vi "2 Simple Time.vi"(11 "Timestamp":string) -> (1 "Error?":bool, 3 "Simple Time":i64)   [LabVIEW 2013]
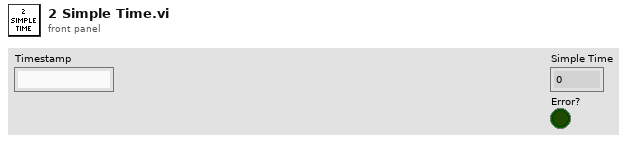
[diagram p1: front panel]
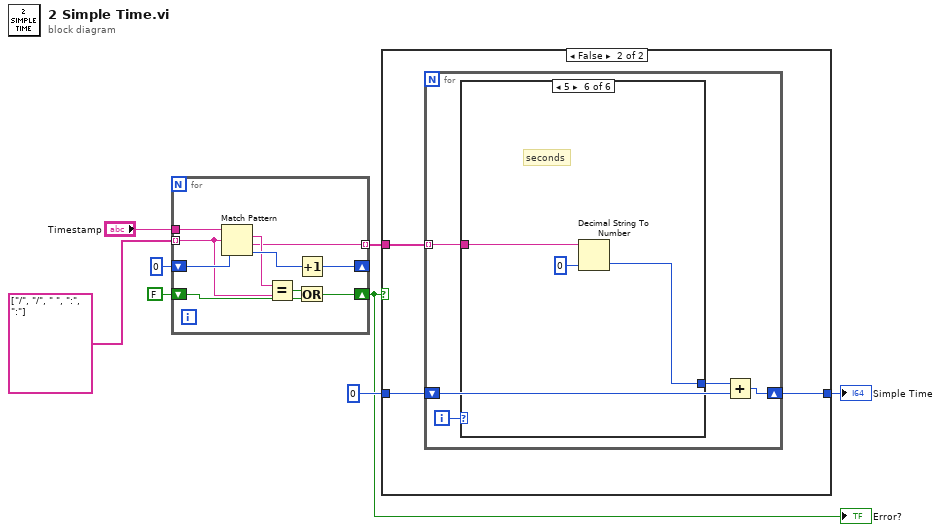
[diagram p0: block diagram]
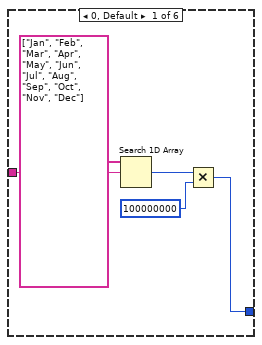
[diagram p3: hidden frame]
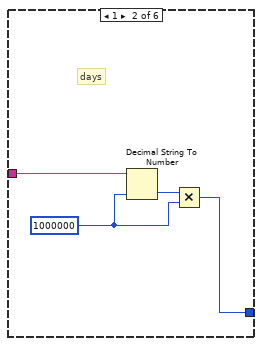
[diagram p4: hidden frame]
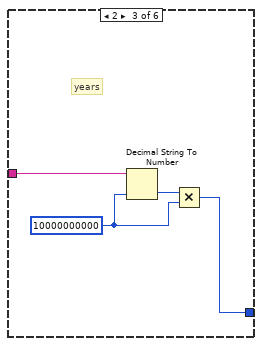
[diagram p5: hidden frame]
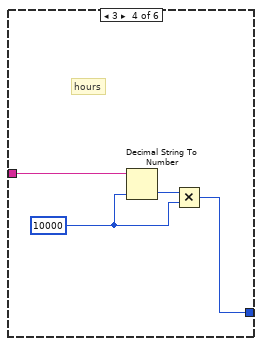
[diagram p6: hidden frame]
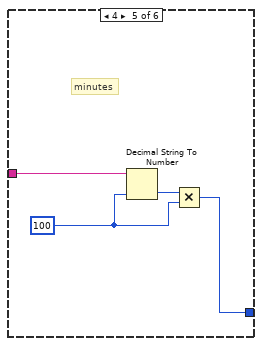
[diagram p7: hidden frame]
diagram:
  n1 = for {
    tunnel: "Timestamp" -> [w18]
    shift-right: [w15] -> _
    shift-left: 0 ("offset past match") -> [w17]
    tunnel: string[] ["/", "/", " ", ":", ":"] -> [w14] mode=indexing
    tunnel: [w12] -> w4 mode=indexing
    shift-right: [w10] -> w1
    shift-left: FALSE -> [w9]
    n2 = Match Pattern(string=w18, regular expression=w14, offset (0)=w17) -> (match substring=w13:string, after substring=w12:string, offset past match=w16:i32)  [unwired: 1 out]
    n3 = Equal?(x=w13, y=w14) -> (x = y?=w11:bool)
    n4 = Increment(x=w16) -> (x+1=w15:i32)
    n5 = Or(x=w11, y=w9) -> (x .or. y?=w10:bool)
  }
  "Error?" <- w1
  n6 = case shown="False" w1 {
    tunnel: w4 -> [_ w22]
    tunnel: [w19 w21] -> w2
    tunnel: i64 0 -> [w19 w20]
    frame True {
      # "Error"
    }
    frame False {
      n7 = for {
        tunnel: w22 -> [w26] mode=indexing
        shift-right: [w24] -> w21
        shift-left: w20 -> [w25]
        i -> [w27]
        n8 = case shown="5" w27 {
          tunnel: w26 -> [w31 w36 w40 w44 w48 w51]
          tunnel: [w28 w33 w37 w41 w45 w49] -> w23
          frame 0, Default {
            n9 = Search 1D Array(1D array=string[] ["Jan", "Feb", "Mar", "Apr", "May", "Jun", "Jul", "Aug", "Sep", "Oct", "Nov", "Dec"], element=w31) -> (index of element=w30:i32)  [unwired: 1 in]
            n10 = Multiply(x=w30, y=i64 100000000) -> (x*y=w28:i64)
          }
          frame 1 {
            w34 = i64 1000000
            # "days"
            n11 = Decimal String To Number(string=w36, default (0L)=w34) -> (number=w35:i64)  [unwired: 1 in, 1 out]
            n12 = Multiply(x=w35, y=w34) -> (x*y=w33:i64)
          }
          frame 2 {
            w38 = i64 10000000000
            # "years"
            n13 = Decimal String To Number(string=w40, default (0L)=w38) -> (number=w39:i64)  [unwired: 1 in, 1 out]
            n14 = Multiply(x=w39, y=w38) -> (x*y=w37:i64)
          }
          frame 3 {
            w42 = i64 10000
            # "hours"
            n15 = Decimal String To Number(string=w44, default (0L)=w42) -> (number=w43:i64)  [unwired: 1 in, 1 out]
            n16 = Multiply(x=w43, y=w42) -> (x*y=w41:i64)
          }
          frame 4 {
            w46 = i64 100
            # "minutes"
            n17 = Decimal String To Number(string=w48, default (0L)=w46) -> (number=w47:i64)  [unwired: 1 in, 1 out]
            n18 = Multiply(x=w47, y=w46) -> (x*y=w45:i64)
          }
          frame 5 {
            # "seconds"
            n19 = Decimal String To Number(string=w51, default (0L)=i64 0) -> (number=w49:i64)  [unwired: 1 in, 1 out]
          }
        }
        n20 = Add(x=w23, y=w25) -> (x+y=w24:i64)
      }
    }
  }
  "Simple Time" <- w2
